vi "Wol_konfig_old_to_new.vi"(8 "error in (no error)":errorcluster, 11 "old Konfig in":T1[](array[typedef]) {"Wolna Wykr num" items=["Brak", "Wykres 1", "Wykres 2", "Wykres 3", "Wykres 4"]}) -> (0 "error out":errorcluster, 3 "new Konfig out":T4[](array[typedef]))   [LabVIEW 2014]
uses:
  Kontrolki/GUI/RejWol_konfig_opis GUI.ctl
  Kontrolki/GUI/RejWol_typ.ctl
  Kontrolki/GUI/RejWol_numer_kanalu.ctl
  Kontrolki/GUI/RejWol_konfig.ctl
  Kontrolki/GUI/Wolna_WykrNum.ctl
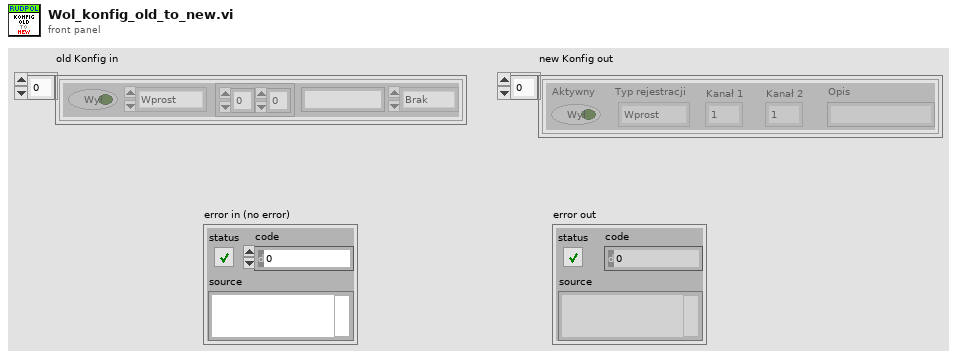
[diagram p1: front panel]
types:
  T1 = typedef "RejWol_konfig.ctl" = cluster{"Typ rejestracji":T2, "Kanały":i32[], "Opis":string, "Aktywny":bool, "Wolna Wykr num":T3}
  T2 = typedef "RejWol_typ.ctl" = enum16{"Wprost", "Moduł", "Kwadrat", "Iloczyn", "Faza"}
  T3 = typedef "Wolna_WykrNum.ctl" = u16
  T4 = typedef "RejWol_konfig_opis GUI.ctl" = cluster{"Typ rejestracji":T2, "Opis":string, "Aktywny":bool, "Kanał 1":T5, "Kanał 2":T5}
  T5 = typedef "RejWol_numer_kanalu.ctl" = enum16{"1", "2", "3", "4", "5", "6", "7", "8"}
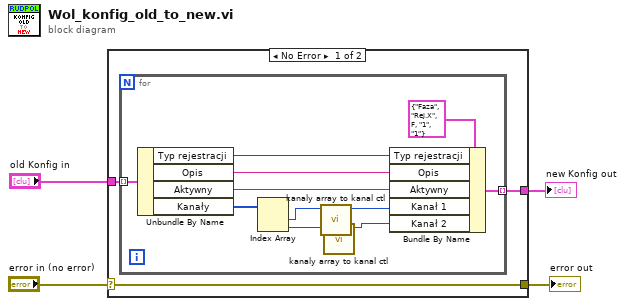
[diagram p0: block diagram]
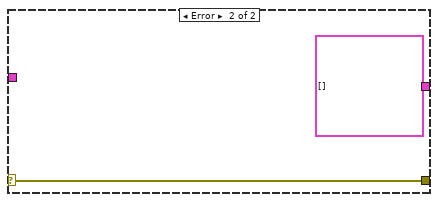
[diagram p2: hidden frame]
diagram:
  n1 = case shown="No Error" "error in (no error)" {
    selector: "error in (no error)" -> [w5 w19]
    tunnel: [w7 T4[] []] -> w4
    tunnel: "old Konfig in" -> [w6 _]
    tunnel: [w5 w19] -> w1
    frame No Error {
      n2 = for {
        tunnel: w6 -> [w18] mode=indexing
        tunnel: [w13] -> w7 mode=indexing
        n3 = Unbundle By Name(w18) -> ("Typ rejestracji"=w16:T2, "Opis"=w15:string, "Aktywny"=w14:bool, "Kanały"=w11:i32[])
        n4 = Index Array(array=w11) -> (element #1=w10:i32, element #2=w8:i32)  [unwired: 2 in]
        n5 = call "kanaly array to kanal ctl.vi"("Chan"=w10) -> ("Kanal"=w12:T5)  [unwired: 10 in]
        n6 = call "kanaly array to kanal ctl.vi"("Chan"=w8) -> ("Kanal"=w9:T5)  [unwired: 10 in]
        n7 = Bundle By Name(cluster=T4 {"Typ rejestracji"=enum."Faza", "Opis"="Rej.X", "Aktywny"=FALSE, "Kanał 1"=enum."1", "Kanał 2"=enum."1"} ("Rejestracja 2a"), "Typ rejestracji"=w16, "Opis"=w15, "Aktywny"=w14, "Kanał 1"=w12, "Kanał 2"=w9) -> (w13:T4)
      }
    }
    frame Error {
    }
  }
  "new Konfig out" <- w4
  "error out" <- w1
